vi "Configure Measurement RRC Filter.vi"(7 "Enable RRC Filter (F: Disable)":bool, 8 "error in (no error)":errorcluster, 9 "Filter Bandwidth (3.84E+6 Hz)":dbl=3840000.0, 10 "Filter Alpha (0.22)":dbl=0.22 format="%#.6g", 11 "VISA resource name":refnum<visa-resource-name>) -> (0 "error out":errorcluster, 3 "VISA resource name out":refnum<visa-resource-name>)   [LabVIEW 2018, in "Agilent MXA Series.lvlib"]
doc: "Configures the RRC Filter."
uses:
  Agilent MXA Series.lvlib
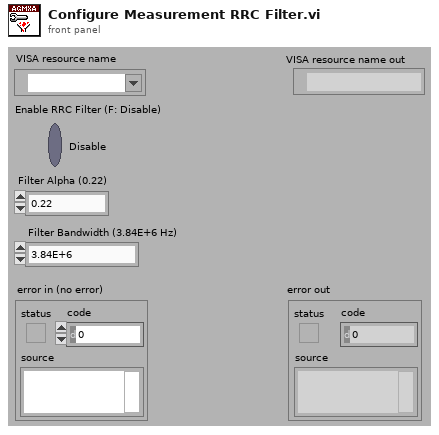
[diagram p1: front panel]
types:
  T1 = typedef "Agilent MXA Series.lvlib/Extended User Data.ctl" = cluster{"Measurement Type":i32, "Agilent MXA/EXA Model":i32}
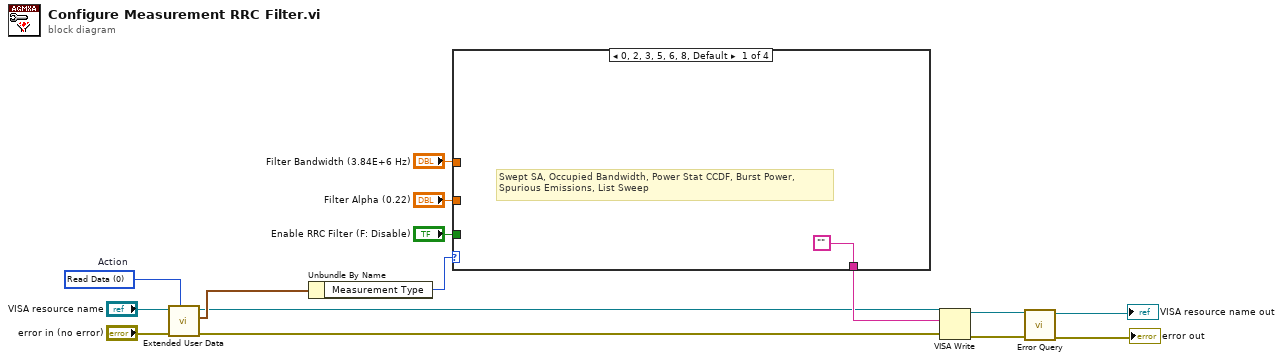
[diagram p0: block diagram]
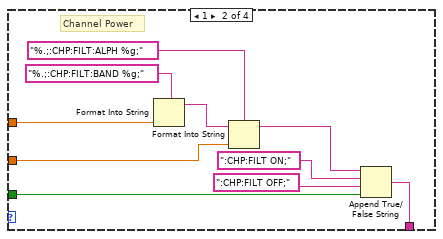
[diagram p2: hidden frame]
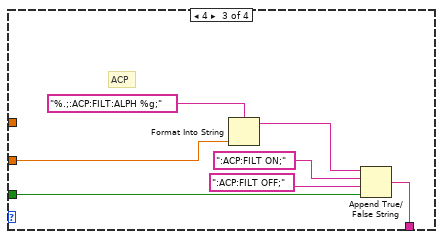
[diagram p3: hidden frame]
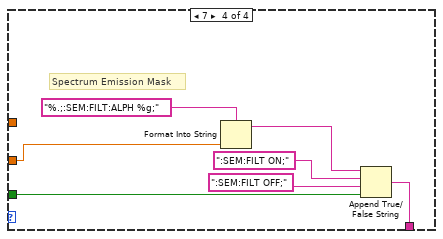
[diagram p4: hidden frame]
diagram:
  w13 = 0 items=["Read Data", "Write Data", "Clear Data", "Clear ALL Data"]  # Action
  n1 = call "Extended User Data.vi"("Action (1:Write Data)"=w13, "Error In (no error)"="error in (no error)", "VISA resource name in"="VISA resource name") -> ("Error Out"=w5:errorcluster, "User Data Out"=w12:T1, "VISA resource name out"=w6:refnum<visa-resource-name>)  [unwired: 6 in]
  n2 = Unbundle By Name(w12) -> ("Measurement Type"=w11:i32)
  n3 = case shown="0, 2, 3, 5, 6, 8, Default" w11 {
    tunnel: "Enable RRC Filter (F: Disable)" -> [_ w21 w31 w38]
    tunnel: "Filter Alpha (0.22)" -> [_ w24 w33 w40]
    tunnel: "Filter Bandwidth (3.84E+6 Hz)" -> [_ w26 _ _]
    tunnel: ["" w17 w27 w34] -> w7
    frame 0, 2, 3, 5, 6, 8, Default {
      # "Swept SA, Occupied Bandwidth, Power Stat CCDF, Burst Power,\nSpurious Emissions, List Sweep"
    }
    frame 1 {
      # "Channel Power"
      n4 = Format Into String(format string="%.;:CHP:FILT:BAND %g;", w26) -> (resulting string=w22:string)  [unwired: 2 in, 1 out]
      n5 = Format Into String(format string="%.;:CHP:FILT:ALPH %g;", initial string=w22, w24) -> (resulting string=w18:string)  [unwired: 1 in, 1 out]
      n6 = Append True/False String(1:w21, 2:":CHP:FILT OFF;" ("false string"), 3:":CHP:FILT ON;" ("true string"), 4:w18) -> (0:w17:string)
    }
    frame 4 {
      # "ACP"
      n7 = Format Into String(format string="%.;:ACP:FILT:ALPH %g;", w33) -> (resulting string=w28:string)  [unwired: 2 in, 1 out]
      n8 = Append True/False String(1:w31, 2:":ACP:FILT OFF;" ("false string"), 3:":ACP:FILT ON;" ("true string"), 4:w28) -> (0:w27:string)
    }
    frame 7 {
      # "Spectrum Emission Mask"
      n9 = Format Into String(format string="%.;:SEM:FILT:ALPH %g;", w40) -> (resulting string=w35:string)  [unwired: 2 in, 1 out]
      n10 = Append True/False String(1:w38, 2:":SEM:FILT OFF;" ("false string"), 3:":SEM:FILT ON;" ("true string"), 4:w35) -> (0:w34:string)
    }
  }
  n11 = VISA Write(VISA resource name=w6, write buffer=w7, error in (no error)=w5) -> (VISA resource name out=w4:refnum<visa-resource-name>, error out=w2:errorcluster)  [unwired: 1 out]
  n12 = call "Error Query.vi"("error in (no error)"=w2, "VISA resource name"=w4) -> ("error out"=→"error out":errorcluster, "VISA resource name out"=→"VISA resource name out":refnum<visa-resource-name>)  [unwired: 6 in, 2 out]
